vi "Auto.vi"() -> ()   [LabVIEW 2020]
uses:
  Global_Variable/Global.vi
  Global_Variable/A180648.vi
  Libraries/S7/S7.lvlib
  <userlib>/_MGI/1D Array/MGI Running Average/MGI Running Average(SGL).vi
panel:
  out "当前曲线":i16
  out "振动NHV-FFT":cluster{"f0":dbl, "df":dbl, "magnitude":dbl[]}[](graph)
  out "振动NVH-Order":cluster{"f0":dbl, "df":dbl, "magnitude":dbl[]}[](graph)
  out "试验项_Event":refnum<user-event>
  out "产品_EVENT":refnum<user-event>
  out "T1+T2":dbl
  out "T2":dbl
  out "T1":dbl
  out "吸收电流":sgl
  out "输出扭矩(大)":sgl
  out "输入扭矩":sgl
  out "当前车速":i32
  out "试验项目":T1(tab)
  out "空载试验":cluster{dbl[], dbl[]}[](graph)
  out "功能试验":cluster{dbl[], dbl[]}[](graph)
  out "力特性试验":cluster{dbl[], dbl[]}[](graph)
  out "电流特性试验":cluster{dbl[], dbl[]}[](graph)
  out "传感器特性试验":cluster{dbl[], dbl[]}[](graph)
  out "逆向空载试验":cluster{dbl[], dbl[]}[](graph)
  out "磨合":cluster{dbl[], dbl[]}[](graph)
  out "振动2NHV-FFT":cluster{"f0":dbl, "df":dbl, "magnitude":dbl[]}[](graph)
  out "振动1NVH-FFT":cluster{"f0":dbl, "df":dbl, "magnitude":dbl[]}[](graph)
  in  "判定结果":bool[][](array[boolean])=[[TRUE]]
  in  "STEP":string
  # "车速0"
  # "车速1"
  # "车速2"
  # "车速3"
  # "车速4"
  # "车速5"
  # "车速0"
  # "车速1"
  # "车速2"
  # "车速3"
  # "车速4"
  # "车速5"
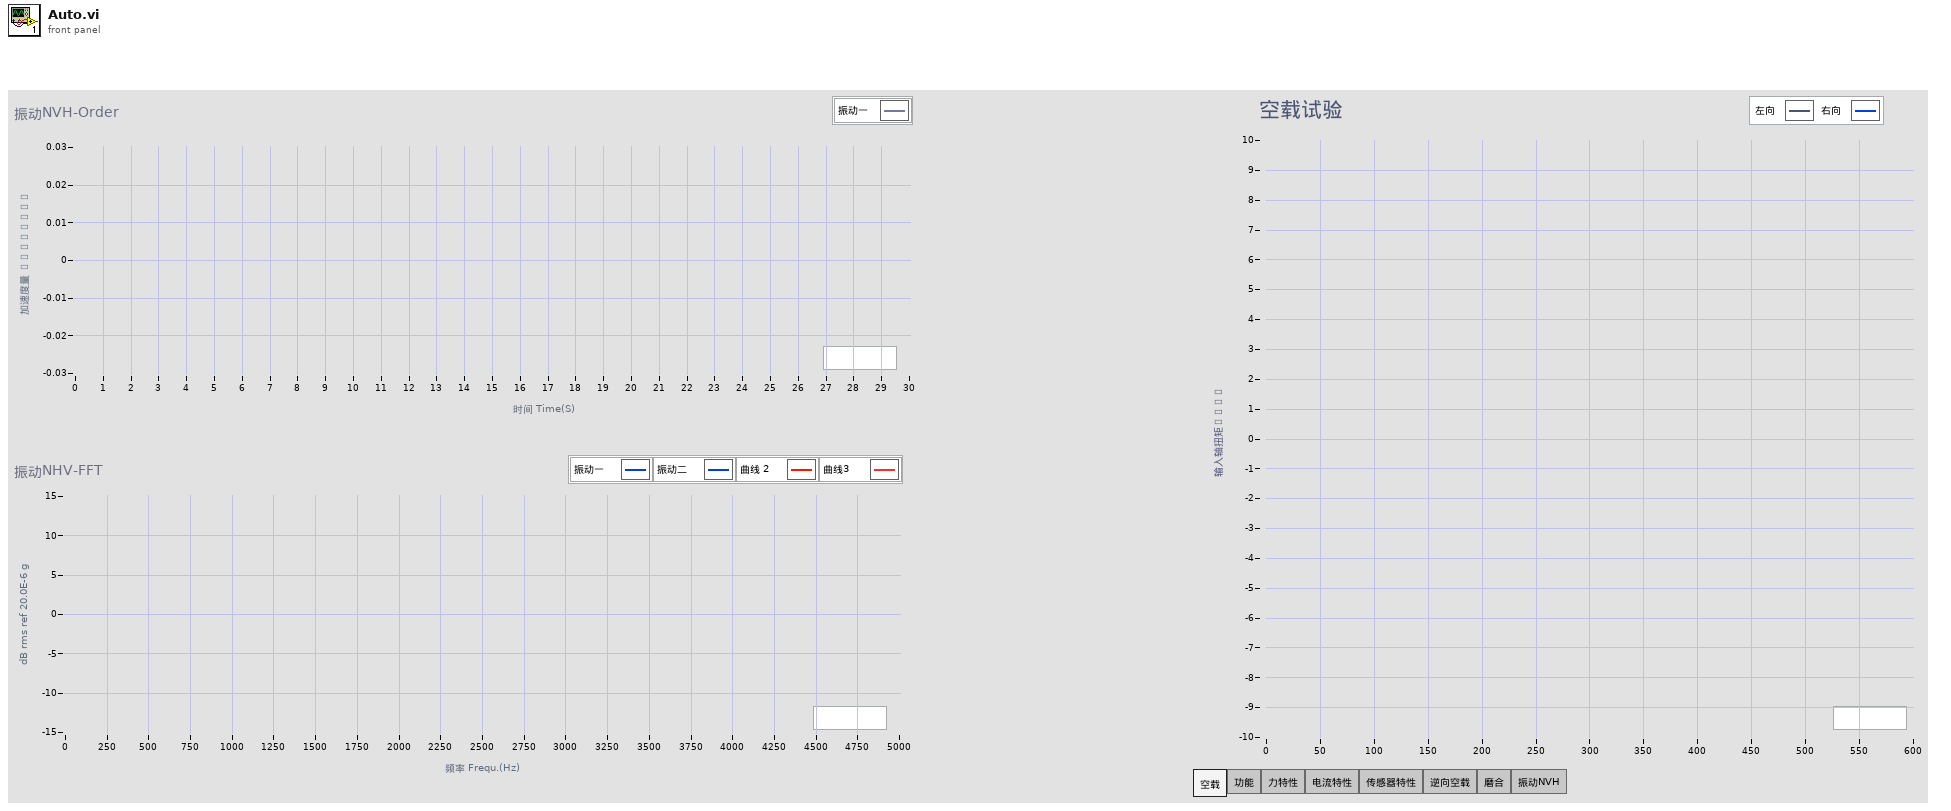
[diagram p1: front panel]
types:
  T1 = enum32{"空载", "功能", "力特性", "电流特性", "传感器特性", "逆向空载", "磨合", "振动NVH"}
  T2 = cluster{"输入轴扭矩":dbl, "输出轴扭矩小量程":dbl, "输出轴扭矩大量程":dbl}
  T3 = enum32{"空载", "功能", "力特性", "电流特性", "传感器特性", "逆向空载", "振动NVH", "磨合", "完成"}
  T4 = typedef "svc_Spectrum Info.ctl" = cluster{"channel name":string, "description":string, "x-axis units":T5, "spectral info":cluster{"spectrum type":T6, "linear/dB":enum16{"linear", "dB"}, "window":u16, "window size":i32, "FFT size":i32}, "engineering units":T7, "custom label":string, "dB reference [EU]":dbl, "peak units":enum16{"rms", "peak", "peak-peak"}, "weighting filter":T8, "spectral density?":bool, "unit label":string, "spectrum skewed?":bool, "complimentary spectrum units":T9}
  T5 = typedef "svc_X-Axis Units.ctl" = u16
  T6 = typedef "svc_Spectrum Type.ctl" = enum16{"FFT Spectrum [complex]", "Amplitude [Magnitude]", "Power [Magnitude^2]", "Cross Spectrum [complex]", "Frequency Response [Complex]"}
  T7 = typedef "svc_Engineering Units Text Ring.ctl" = u16
  T8 = typedef "svc_Weighting Filter Text Ring.ctl" = u16
  T9 = typedef "svc_Complimentary Spectrum Units.ctl" = enum16{"none", "radians", "degrees", "cycles", "imaginary"}
  T10 = cluster{"振动1频率检测段1范围":cluster{"单位":string, "下限":dbl, "上限":dbl}, "振动1频率检测段2范围":cluster{"单位":string, "下限":dbl, "上限":dbl}, "振动1频率检测段3范围":cluster{"单位":string, "下限":dbl, "上限":dbl}, "振动1频率检测段4范围":cluster{"单位":string, "下限":dbl, "上限":dbl}, "振动1频率检测段5范围":cluster{"单位":string, "下限":dbl, "上限":dbl}}
  T11 = cluster{"振动1频率检测段1振幅":cluster{"单位":string, "下限":dbl, "上限":dbl}, "振动1频率检测段2振幅":cluster{"单位":string, "下限":dbl, "上限":dbl}, "振动1频率检测段3振幅":cluster{"单位":string, "下限":dbl, "上限":dbl}, "振动1频率检测段4振幅":cluster{"单位":string, "下限":dbl, "上限":dbl}, "振动1频率检测段5振幅":cluster{"单位":string, "下限":dbl, "上限":dbl}}
  T12 = cluster{"输入旋转位移":sgl, "输入移载位移":sgl, "工装移载位移":sgl, "输入编码位移":sgl, "输入扭矩":sgl, "输出扭矩(小)":sgl, "输出扭矩(大)":sgl, "吸收电流":sgl, "Factorysensor":sgl, "输出轴旋转角度":sgl, "输出轴移栽位移":sgl, "Factorysensor2":sgl}
  T13 = typedef "lveventtype.ctl" = enum32{"Null", "Timeout", "Annotation Menu Selection", "Annotation Menu Selection?", "App Instance Close", "App Instance Close?", "Autoscale Range Change", "Bookmark Info Change", "Cell Edit", "Cell Edit?", "Cursor Grab", "Cursor Grab?", "Cursor Menu Selection", "Cursor Menu Selection?", "Cursor Move", "Cursor Release", "Data Change", "Direction Change", "Display State Change", "Drag Ended", "Drag Enter", "Drag Leave", "Drag Over", "Drag Source Update", "Drag Starting", "Drag Starting?", "Drop", "Exec State Change", "Key Down", "Key Down?", "Key Repeat", "Key Repeat?", "Key Up", "Listbox Double Click", "Menu Activation?", "Menu Selection (App)", "Menu Selection? (App)", "Menu Selection (User)", "Mouse Down", "Mouse Down?", "Mouse Enter", "Mouse Leave", "Mouse Move", "Mouse Up", "Mouse Wheel", "NI Security User Change (App)", "Pane Size", "Panel Close", "Panel Close?", "Panel Resize", "Plot Attribute Change", "Scale Range Change", "Shortcut Menu Activation?", "Shortcut Menu Selection (App)", "Shortcut Menu Selection? (App)", "Shortcut Menu Selection (User)", "Tree Double Click", "Tree Drag", "Tree Drag?", "Tree Drop", "Tree Drop?", "Tree Item Close", "Tree Item Close?", "Tree Item Open", "Tree Item Open?", "User Event", "Value Change"}
  T14 = typedef "LVPoint32TypeDef.ctl" = cluster{"Horizontal":i32, "Vertical":i32}
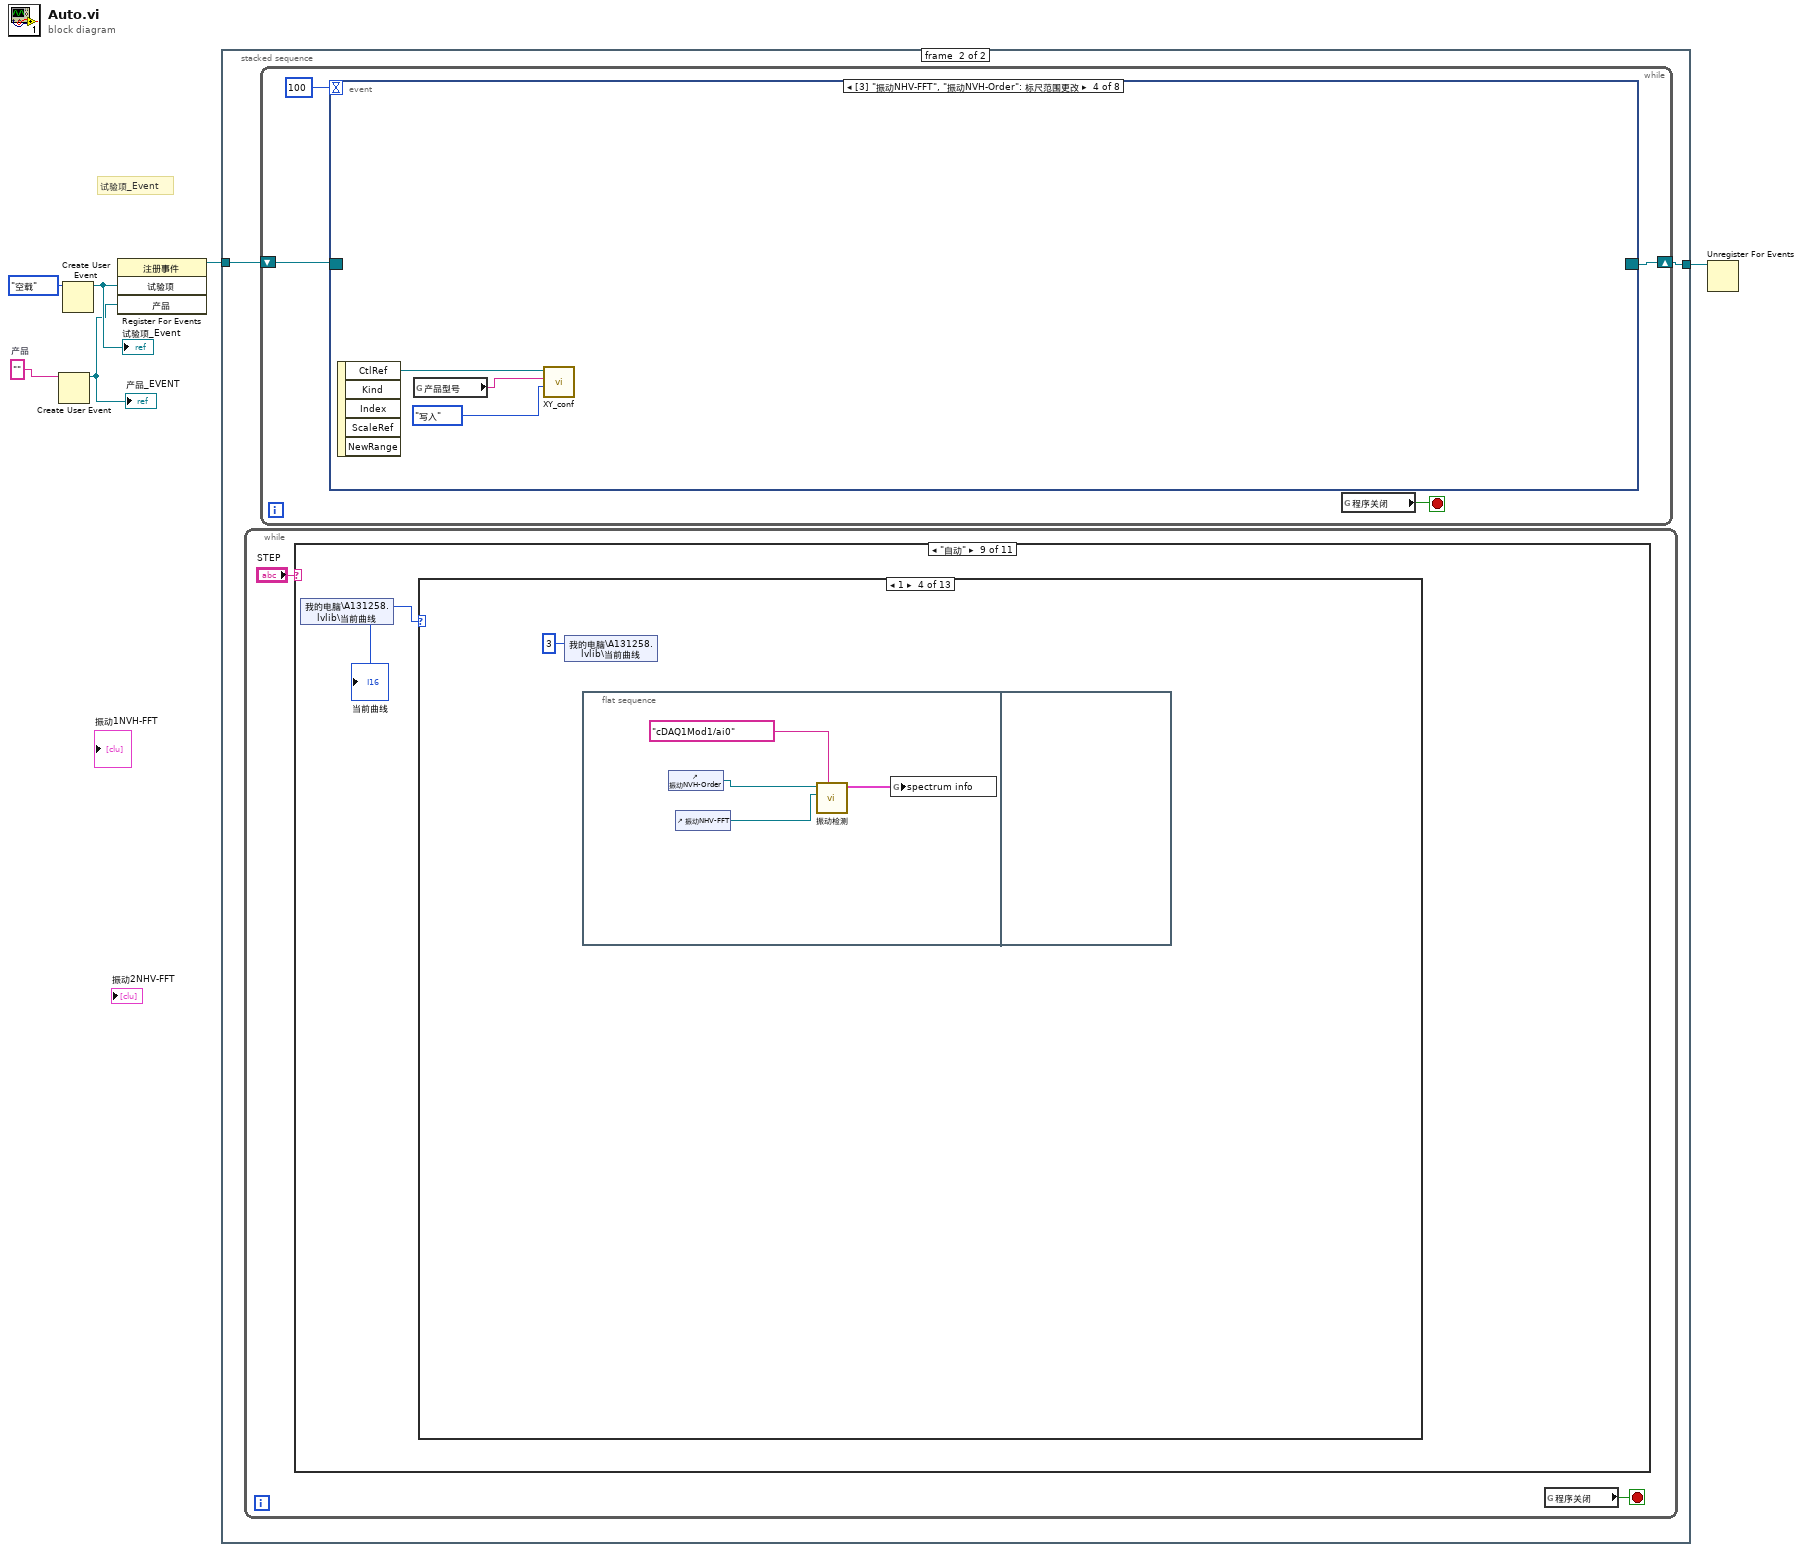
[diagram p0: block diagram]
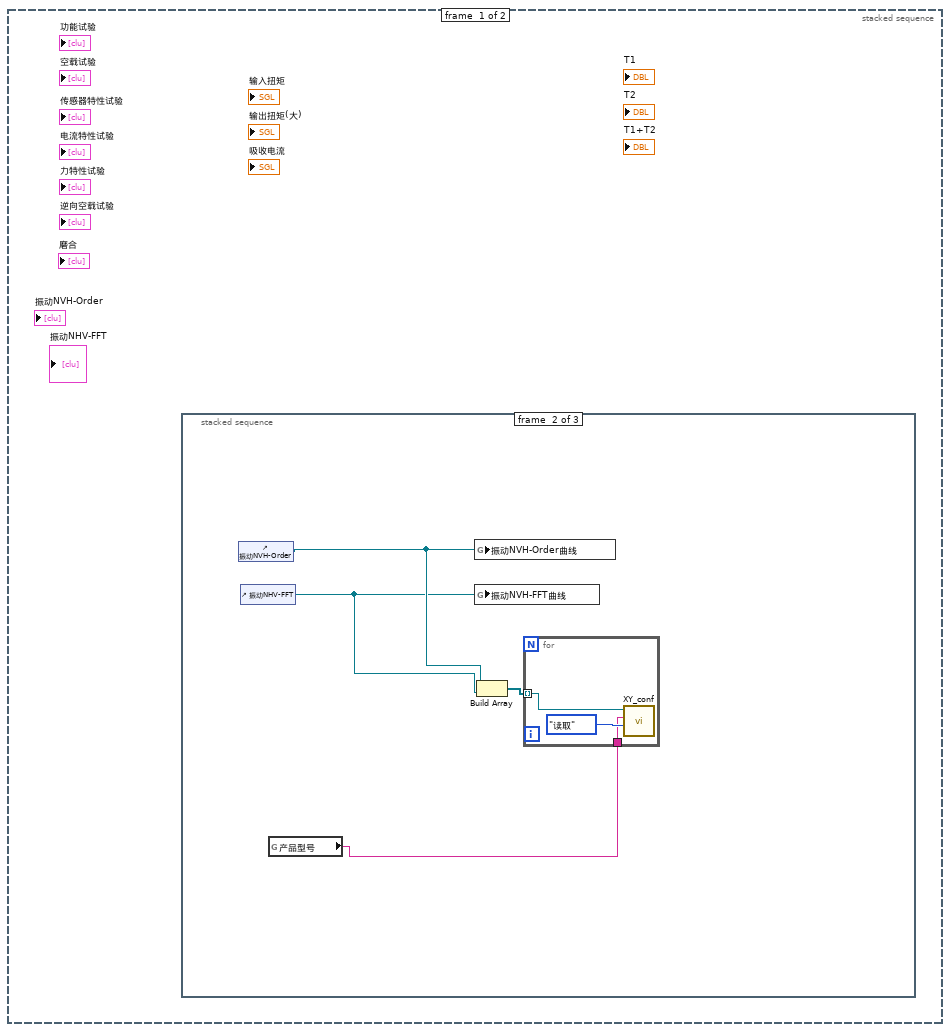
[diagram p2: hidden frame]
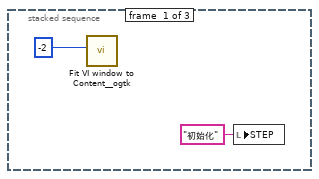
[diagram p3: hidden frame]
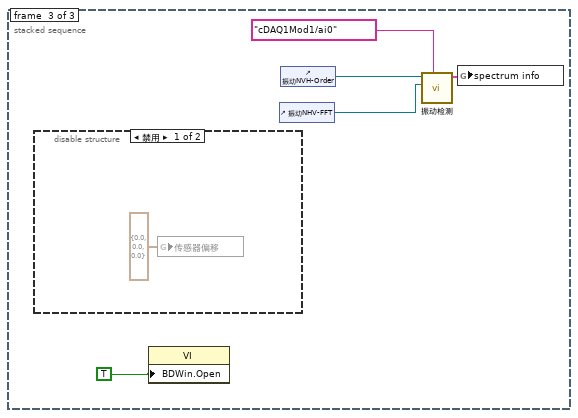
[diagram p4: hidden frame]
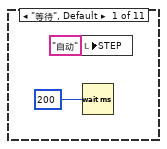
[diagram p6: hidden frame]
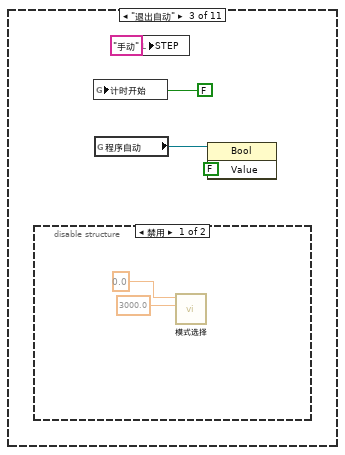
[diagram p8: hidden frame]
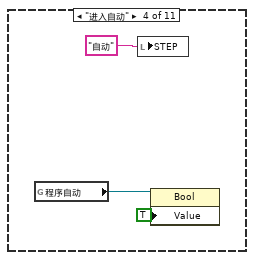
[diagram p10: hidden frame]
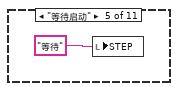
[diagram p11: hidden frame]
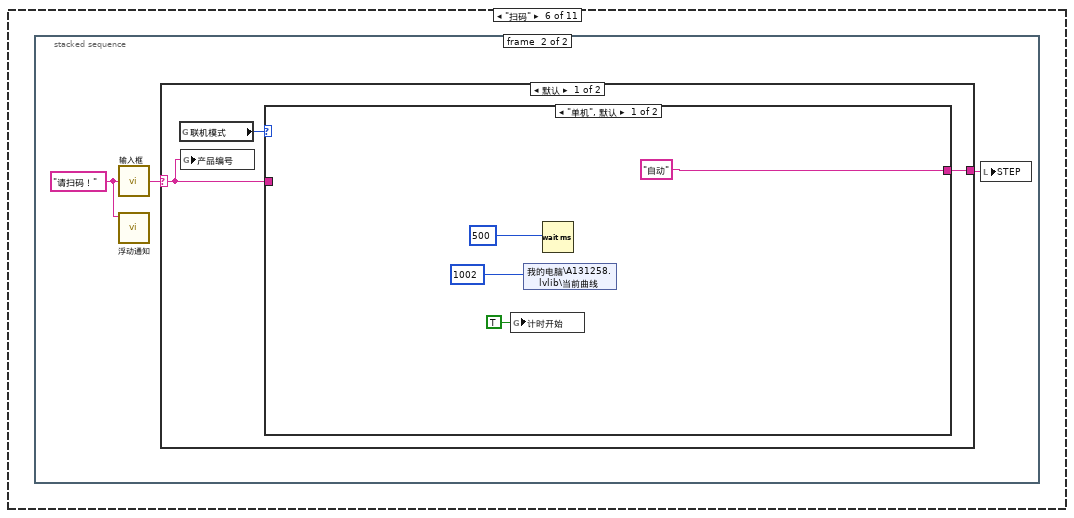
[diagram p12: hidden frame]
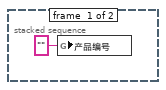
[diagram p13: hidden frame]
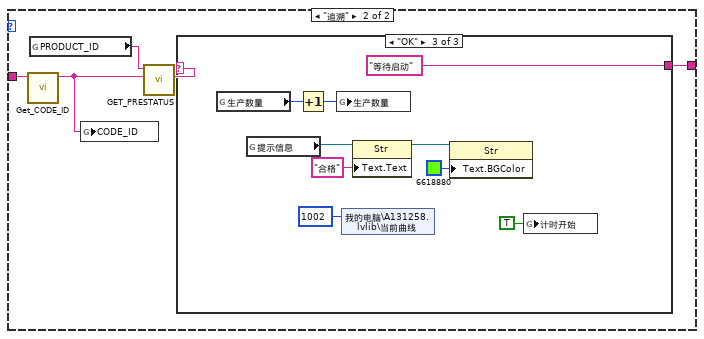
[diagram p14: hidden frame]
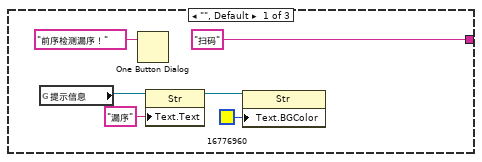
[diagram p15: hidden frame]
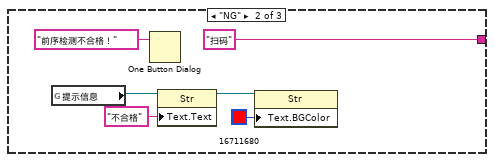
[diagram p16: hidden frame]
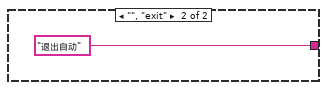
[diagram p17: hidden frame]
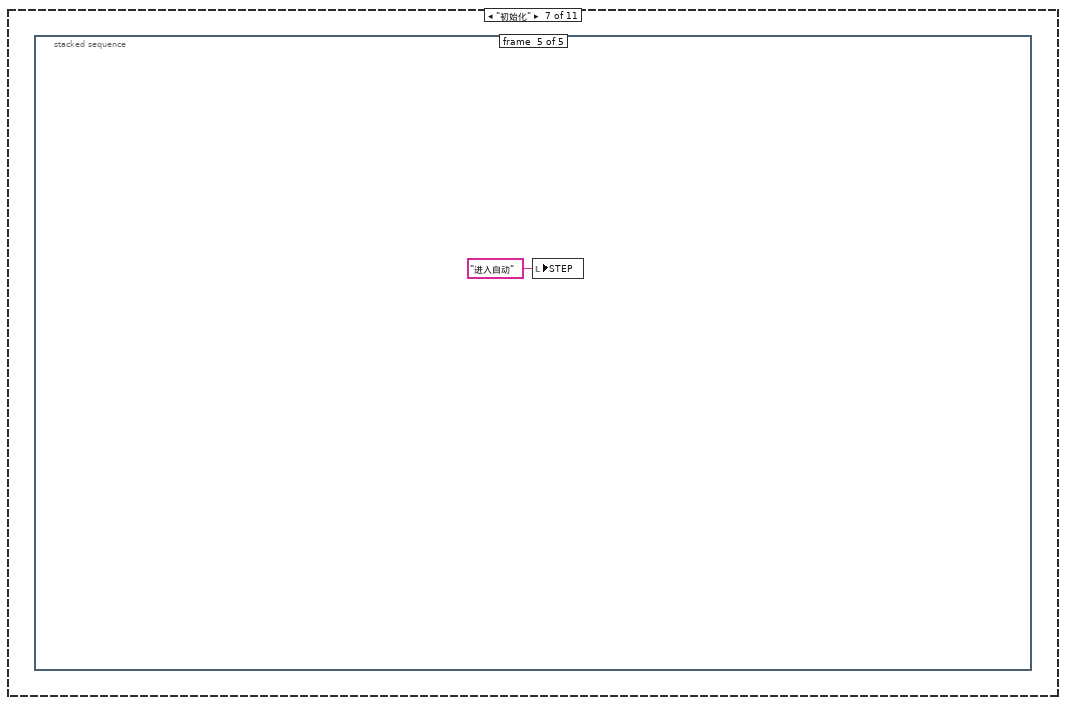
[diagram p18: hidden frame]
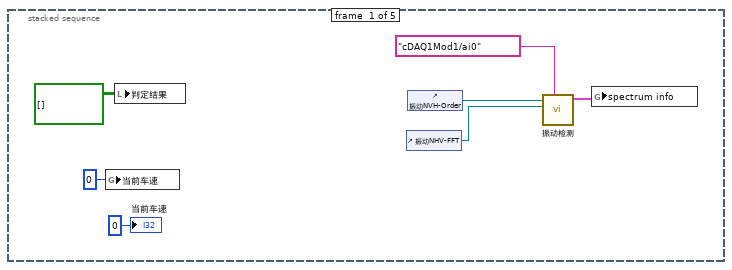
[diagram p19: hidden frame]
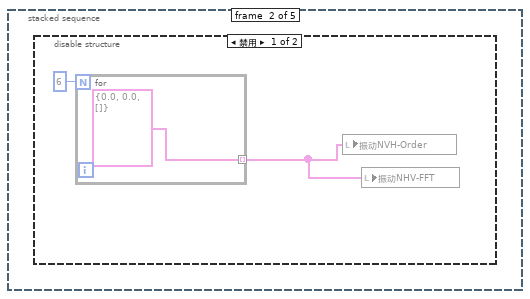
[diagram p20: hidden frame]
diagram:
  w2 = ""  # 产品
  # "试验项_Event"
  n1 = Create User Event(user event datatype=w2) -> (user event=w1:refnum<user-event>)  [unwired: 1 in, 1 out]
  "产品_EVENT" <- w1
  n2 = Create User Event(user event datatype=T1."空载" ("试验项")) -> (user event=w4:refnum<user-event>)  [unwired: 1 in, 1 out]
  "试验项_Event" <- w4
  n3 = register-events(w4, w1) -> (reference out=w5:refnum<event-registration>)  [unwired: 2 in, 1 out]
  n4 = stacked-sequence {
    tunnel: w5 -> [_ w23]
    tunnel: [_ w22] -> w3
    frame #0 {
      n5 = stacked-sequence {
        frame #0 {
          n6 = call <userlib>:"Fit VI window to Content__ogtk.vi"("border spacing (2 px)"=-2) -> ()  [unwired: 5 in, 2 out]
          n7 = local write "STEP"("初始化" ("STEP")) -> ()
        }
        frame #1 {
          n8 = control-ref of="振动NVH-Order"() -> (w10:refnum<vi>)
          n9 = control-ref of="振动NHV-FFT"() -> (w9:refnum<vi>)
          n10 = global read "Global.vi" "产品型号"() -> (w11:string)
          n11 = global write "A180648.vi" "振动NVH-Order曲线"(w10) -> ()
          n12 = global write "A180648.vi" "振动NVH-FFT曲线"(w9) -> ()
          n13 = Build Array(w10, w9) -> (w12:refnum<vi>[])
          n14 = for {
            tunnel: w12 -> [w13] mode=indexing
            tunnel: w11 -> [w14]
            n15 = call "XY_conf.vi"("方式"=enum16{"写入", "读取"}."读取", "产品"=w14, "XY图引用"=w13) -> ()  [unwired: 4 in, 1 out]
          }
        }
        frame #2 {
          n16 = disable-structure shown="禁用" {
            frame Disabled {
              n17 = global write "传感器偏移.vi" "传感器偏移"(T2 {"输入轴扭矩"=0.0, "输出轴扭矩小量程"=0.0, "输出轴扭矩大量程"=0.0} ("传感器偏移")) -> ()
            }
            frame Enabled {
            }
          }
          n18 = property class="VI"("BDWin.Open"=TRUE ("程序框图窗口:打开")) -> ()  [unwired: 2 in, 2 out]
          n19 = control-ref of="振动NHV-FFT"() -> (w17:refnum<vi>)
          n20 = control-ref of="振动NVH-Order"() -> (w18:refnum<vi>)
          n21 = call "振动检测.vi"("通道输入"=tag "cDAQ1Mod1/ai0" ("DAQmx物理通道"), "WFGraph引用句柄FFT"=w17, "WFGraph引用句柄Order"=w18) -> ("spectrum info"=w19:T4[])  [unwired: 7 in, 1 out]
          n22 = global write "Global.vi" "spectrum info"(w19) -> ()
        }
      }
    }
    frame #1 {
      n23 = while {
        stop <- w25 stop-if-true
        n24 = case shown="\"自动\"" "STEP" {
          frame "等待", Default {
            n25 = local write "STEP"("自动" ("STEP")) -> ()
            n26 = Wait (ms)(milliseconds to wait=u32 200 ("等待时间（毫秒）")) -> ()  [unwired: 1 out]
          }
          frame "手动" {
          }
          frame "退出自动" {
            n27 = disable-structure shown="禁用" {
              frame Disabled {
                n28 = call-poly "模式选择.vi"("Max Torque"=sgl 3000.0, "Velocity"=sgl 0.0) -> ()  [unwired: 9 in, 1 out]
              }
              frame Enabled {
              }
            }
            n29 = global write "Global.vi" "计时开始"(FALSE ("计时开始")) -> ()
            n30 = global read "Global.vi" "程序自动"() -> (w29:refnum<vi>)
            n31 = local write "STEP"("手动" ("STEP")) -> ()
            n32 = property class="Bool"(reference=w29, "Value"=FALSE) -> ()  [unwired: 1 in, 2 out]
          }
          frame "进入自动" {
            n33 = global read "Global.vi" "程序自动"() -> (w35:refnum<vi>)
            n34 = local write "STEP"("自动" ("STEP")) -> ()
            n35 = property class="Bool"(reference=w35, "Value"=TRUE) -> ()  [unwired: 1 in, 2 out]
          }
          frame "等待启动" {
            n36 = local write "STEP"("等待" ("STEP")) -> ()
          }
          frame "扫码" {
            n37 = stacked-sequence {
              frame #0 {
                n38 = global write "Global.vi" "产品编号"("" ("产品编号")) -> ()
              }
              frame #1 {
                w40 = "请扫码！" ("提示信息")
                n39 = call "输入框.vi"("提示信息"=w40) -> ("条形码输出"=w41:string)
                n40 = call "浮动通知.vi"("通知内容"=w40) -> ()  [unwired: 11 in]
                n41 = case shown="默认" w41 {
                  selector: w41 -> [w43 _]
                  tunnel: [w44 "退出自动" ("State(s) in Front (\"\")")] -> w39
                  frame Default {
                    n42 = global read "Global.vi" "联机模式"() -> (w42:enum16{"单机", "追溯"})
                    n43 = global write "Global.vi" "产品编号"(w43) -> ()
                    n44 = case shown="\"单机\", 默认" w42 {
                      tunnel: ["自动" ("State(s) in Front (\"\")") w53] -> w44
                      tunnel: w43 -> [_ w51]
                      frame "单机", Default {
                        n45 = global write "Global.vi" "计时开始"(TRUE ("计时开始")) -> ()
                        n46 = shared-variable "我的电脑\\A131258.lvlib\\当前曲线"(i16 1002 ("当前曲线")) -> ()  [unwired: 1 in, 1 out]
                        n47 = Wait (ms)(milliseconds to wait=u32 500 ("等待时间（毫秒）")) -> ()  [unwired: 1 out]
                      }
                      frame "追溯" {
                        n48 = call "Get_CODE_ID.vi"("CODE_SENSOR"=w51) -> ("CODE_ID"=w50:string)  [unwired: 10 in]
                        n49 = global read "追溯Global.vi" "PRODUCT_ID"() -> (w52:string)
                        n50 = global write "追溯Global.vi" "CODE_ID"(w50) -> ()
                        n51 = call "GET_PRESTATUS.vi"("CODE_ID"=w50, "PRODUCT_ID"=w52) -> ("字符串"=w49:string)  [unwired: 8 in, 1 out]
                        n52 = case shown="\"OK\"" w49 {
                          tunnel: ["扫码" ("State(s) in Front (\"\")") "扫码" ("State(s) in Front (\"\")") "等待启动" ("State(s) in Front (\"\")")] -> w53
                          frame "", Default {
                            n53 = global read "Global.vi" "提示信息"() -> (w57:refnum<vi>)
                            n54 = One Button Dialog(message="前序检测漏序！" ("消息")) -> ()  [unwired: 1 in, 1 out]
                            n55 = property class="Str"(reference=w57, "Text.Text"="漏序" ("文本.文本")) -> (reference out=w55:refnum<vi>)  [unwired: 1 in, 1 out]
                            n56 = property class="Str"(reference=w55, "Text.BGColor"=u32 16776960 ("文本.文本颜色:背景色")) -> ()  [unwired: 1 in, 2 out]
                          }
                          frame "NG" {
                            n57 = global read "Global.vi" "提示信息"() -> (w63:refnum<vi>)
                            n58 = One Button Dialog(message="前序检测不合格！" ("消息")) -> ()  [unwired: 1 in, 1 out]
                            n59 = property class="Str"(reference=w63, "Text.Text"="不合格" ("文本.文本")) -> (reference out=w61:refnum<vi>)  [unwired: 1 in, 1 out]
                            n60 = property class="Str"(reference=w61, "Text.BGColor"=u32 16711680 ("文本.文本颜色:背景色")) -> ()  [unwired: 1 in, 2 out]
                          }
                          frame "OK" {
                            n61 = global read "Global.vi" "生产数量"() -> (w72:i32)
                            n62 = global read "Global.vi" "提示信息"() -> (w71:refnum<vi>)
                            n63 = Increment(x=w72) -> (x+1=w73:i32)
                            n64 = global write "Global.vi" "生产数量"(w73) -> ()
                            n65 = shared-variable "我的电脑\\A131258.lvlib\\当前曲线"(i16 1002 ("当前曲线")) -> ()  [unwired: 1 in, 1 out]
                            n66 = property class="Str"(reference=w71, "Text.Text"="合格" ("文本.文本")) -> (reference out=w69:refnum<vi>)  [unwired: 1 in, 1 out]
                            n67 = property class="Str"(reference=w69, "Text.BGColor"=u32 6618880 ("文本.文本颜色:背景色")) -> ()  [unwired: 1 in, 2 out]
                            n68 = global write "Global.vi" "计时开始"(TRUE ("计时开始")) -> ()
                          }
                        }
                      }
                    }
                  }
                  frame "", "exit" {
                  }
                }
                n69 = local write "STEP"(w39) -> ()
              }
            }
          }
          frame "初始化" {
            n70 = stacked-sequence {
              frame #0 {
                n71 = global write "A180648.vi" "当前车速"(u16 0 ("当前车速")) -> ()
                n72 = local write "判定结果"(bool[][] [] ("判定结果")) -> ()
                n73 = control-ref of="振动NHV-FFT"() -> (w78:refnum<vi>)
                n74 = control-ref of="振动NVH-Order"() -> (w79:refnum<vi>)
                n75 = call "振动检测.vi"("通道输入"=tag "cDAQ1Mod1/ai0" ("DAQmx物理通道"), "WFGraph引用句柄FFT"=w78, "WFGraph引用句柄Order"=w79) -> ("spectrum info"=w77:T4[])  [unwired: 7 in, 1 out]
                n76 = global write "Global.vi" "spectrum info"(w77) -> ()
                "当前车速" <- 0 ("当前车速")
              }
              frame #1 {
                n77 = disable-structure shown="禁用" {
                  frame Disabled {
                    n78 = for {
                      N: 6 -> [_]
                      tunnel: [cluster{"f0":dbl, "df":dbl, "magnitude":dbl[]} {"f0"=0.0, "df"=0.0, "magnitude"=[]} ("power spectrum [dB EU]")] -> w83 mode=indexing
                    }
                    n79 = local write "振动NVH-Order"(w83) -> ()
                    n80 = local write "振动NHV-FFT"(w83) -> ()
                  }
                  frame Enabled {
                  }
                }
              }
              frame #2 {
                n81 = global read "Global.vi" "Result"() -> (w88:refnum<vi>)
                n82 = property class="Tbl"(reference=w88, "Value"=string[][] []) -> (reference out=w89:refnum<vi>, error out=w90:errorcluster)  [unwired: 1 in]
                n83 = property class="Tbl"(reference=w89, error in=w90, "Row Headers[]"=string[] [] ("列首字符串[]")) -> ()  [unwired: 2 out]
              }
              frame #3 {
                w91 = 1 ("维数大小")
                n84 = Initialize Array(" " ("字符串"), w91, w91, w91) -> (w94:string[][][])
                n85 = global write "A180648.vi" "检测结果"(w94) -> ()
                n86 = global write "A180648.vi" "当前检测项"(T3."空载" ("当前检测项")) -> ()
              }
              frame #4 {
                n87 = local write "STEP"("进入自动" ("STEP")) -> ()
              }
            }
          }
          frame "判定" {
            n88 = stacked-sequence {
              frame #0 {
                n89 = local read "振动NHV-FFT"() -> (w98:cluster{"f0":dbl, "df":dbl, "magnitude":dbl[]}[])
                n90 = global read "判定参数.vi" "振动判定范围"() -> (w110:T10)
                n91 = global read "判定参数.vi" "振动判定"() -> (w109:T11)
                n92 = global read "Global.vi" "Result"() -> (w104:refnum<vi>)
                n93 = call "振动判定.vi"("Result"=w104, "振动判定"=w109, "振动判定范围"=w110, "FFT"=w98) -> ("FFT 2"=w97:cluster{"f0":dbl, "df":dbl, "magnitude":dbl[]}[], "OK？"=w99:bool)  [unwired: 6 in]
                n94 = global read "A180648.vi" "LED-振动NVH"() -> (w105:refnum<vi>)
                n95 = local read "判定结果"() -> (w100:bool[][])
                n96 = Select(t=cluster{u32, u32}[] [{6618880, 6618880}, {6618880, 6618880}, {6618880, 6618880}, {6618880, 6618880}] ("颜色[4]"), s=w99, f=cluster{u32, u32}[] [{16711680, 16711680}, {16711680, 16711680}, {16711680, 16711680}, {16711680, 16711680}] ("颜色[4]")) -> (s? t:f=w107:cluster{u32, u32}[])
                n97 = Build Array(TRUE, w99) -> (w103:bool[])
                n98 = local write "振动NHV-FFT"(w97) -> ()
                n99 = property class="Bool"(reference=w105, "Colors [4]"=w107) -> ()  [unwired: 1 in, 2 out]
                n100 = Build Array (concatenate)(w100, w103) -> (w101:bool[][])
                n101 = local write "判定结果"(w101) -> ()
                n102 = case shown="假" w99 {
                  frame False {
                    n103 = shared-variable "我的电脑\\A131258.lvlib\\上位机测试结果"(u16 200 ("上位机测试结果")) -> ()  [unwired: 1 in, 1 out]
                  }
                  frame True {
                    n104 = shared-variable "我的电脑\\A131258.lvlib\\上位机测试结果"(u16 100 ("上位机测试结果")) -> ()  [unwired: 1 in, 1 out]
                  }
                }
                n105 = shared-variable "我的电脑\\A131258.lvlib\\当前曲线"(i16 4 ("当前曲线")) -> ()  [unwired: 1 in, 1 out]
              }
              frame #1 {
                n106 = local write "STEP"("报表" ("STEP")) -> ()
              }
            }
          }
          frame "自动" {
            n107 = shared-variable "我的电脑\\A131258.lvlib\\当前曲线"() -> (w114:i16)  [unwired: 1 in, 1 out]
            "当前曲线" <- w114
            n108 = case shown="1" w114 {
              frame -128 {
                n109 = disable-structure shown="禁用" {
                  disable-tunnel: [w118 _] -> w115
                  frame Disabled {
                    n110 = call-poly "模式选择.vi"() -> ("error out"=w118:errorcluster)  [unwired: 11 in]
                  }
                  frame Enabled {
                  }
                }
                n111 = global write "Global.vi" "计时开始"(FALSE ("计时开始")) -> ()
                n112 = disable-structure shown="禁用" {
                  disable-tunnel: w115 -> [w119 _]
                  frame Disabled {
                    n113 = call "SetActualPosition.vi"("error in (no error)"=w119) -> ()  [unwired: 10 in, 1 out]
                  }
                  frame Enabled {
                  }
                }
                n114 = call "浮动通知.vi"("通知内容"="复位中……" ("Status")) -> ()  [unwired: 11 in]
              }
              frame Default {
              }
              frame 0 {
                n115 = global write "Global.vi" "计时开始"(FALSE ("计时开始")) -> ()
                n116 = call "浮动通知.vi"("通知内容"="手动状态！" ("Status")) -> ()  [unwired: 11 in]
              }
              frame 1 {
                n117 = shared-variable "我的电脑\\A131258.lvlib\\当前曲线"(i16 3 ("当前曲线")) -> ()  [unwired: 1 in, 1 out]
                n118 = flat-sequence {
                  frame #0 {
                    n119 = control-ref of="振动NVH-Order"() -> (w124:refnum<vi>)
                    n120 = control-ref of="振动NHV-FFT"() -> (w123:refnum<vi>)
                    n121 = call "振动检测.vi"("通道输入"=tag "cDAQ1Mod1/ai0" ("DAQmx物理通道"), "WFGraph引用句柄FFT"=w123, "WFGraph引用句柄Order"=w124) -> ("spectrum info"=w126:T4[])  [unwired: 7 in, 1 out]
                    n122 = global write "Global1.vi" "spectrum info"(w126) -> ()
                  }
                  frame #1 {
                  }
                }
              }
              frame 2 {
                n123 = for {
                  N: 6 -> [_]
                  tunnel: [cluster{dbl[], dbl[]} {[], []}] -> _ mode=indexing
                  tunnel: [cluster{"f0":dbl, "df":dbl, "magnitude":dbl[]} {"f0"=0.0, "df"=0.0, "magnitude"=[]} ("power spectrum [dB EU]")] -> w133 mode=indexing
                }
                n124 = global read "Global.vi" "Result"() -> (w129:refnum<vi>)
                n125 = property class="Tbl"(reference=w129, "Value"=string[][] []) -> (reference out=w130:refnum<vi>, error out=w131:errorcluster)  [unwired: 1 in]
                n126 = local write "振动NVH-Order"(w133) -> ()
                n127 = local write "振动NHV-FFT"(w133) -> ()
                n128 = property class="Tbl"(reference=w130, error in=w131, "Row Headers[]"=string[] [] ("列首字符串[]")) -> ()  [unwired: 2 out]
              }
              frame 3 {
                n129 = local write "STEP"("判定" ("STEP")) -> ()
              }
              frame 5 {
                n130 = global write "Global.vi" "计时开始"(FALSE ("计时开始")) -> ()
              }
              frame 8 {
                n131 = call "浮动通知.vi"("通知内容"="程序停止！" ("Status")) -> ()  [unwired: 11 in]
              }
              frame 100 {
                n132 = call "浮动通知.vi"("通知内容"="请放入产品后按启动夹紧产品！" ("Status")) -> ()  [unwired: 11 in]
              }
              frame 122 {
                n133 = disable-structure shown="禁用" {
                  frame Disabled {
                    w142 = 4 ("Averaging Size")
                    n134 = call "传感器数据.vi"() -> ("传感器读数"=w149:T12)  [unwired: 10 in, 1 out]
                    n135 = Unbundle By Name(w149) -> ("输入编码位移"=w147:sgl, "输入扭矩"=w140:sgl, "输出扭矩(大)"=w144:sgl)
                    n136 = local read item#-1() -> (w141)
                    n137 = call-poly <userlib>:"MGI Running Average.vi"("Averaging Size"=w142, "Initialize? (F)"=w141, "Value"=w147) -> ("Average"=w146:sgl)  [unwired: 8 in]
                    n138 = call-poly <userlib>:"MGI Running Average.vi"("Averaging Size"=w142, "Initialize? (F)"=w141, "Value"=w140) -> ("Average"=w145:sgl)  [unwired: 8 in]
                    n139 = call-poly <userlib>:"MGI Running Average.vi"("Averaging Size"=w142, "Initialize? (F)"=w141, "Value"=w144) -> ("Average"=w143:sgl)  [unwired: 8 in]
                    n140 = Greater Or Equal To 0?(x=w146) -> (x >= 0?=w148:bool)
                    n141 = case shown="真" w148 {
                      tunnel: w145 -> [_ w167]
                      tunnel: w143 -> [_ w164]
                      tunnel: w146 -> [_ w163]
                      frame False {
                      }
                      frame True {
                        n142 = control-ref of="功能试验"() -> (w166:refnum<vi>)
                        n143 = call "曲线采集.vi"("曲线引用"=w166, "曲线索引"=0, "X"=w163, "Y"=w167) -> ("错误输出"=w162:errorcluster)  [unwired: 10 in, 1 out]
                        n144 = call "曲线采集.vi"("曲线引用"=w166, "曲线索引"=2, "X"=w163, "Y"=w164) -> ()  [unwired: 10 in, 2 out]
                        n145 = Unbundle By Name(w162) -> ("status"=w161:bool)
                        n146 = local write item#-1(w161) -> ()
                      }
                    }
                    n147 = case shown="真" w141 {
                      frame False {
                      }
                      frame True {
                        n148 = control-ref of="振动1NVH-FFT"() -> (w151:refnum<vi>)
                        n149 = control-ref of="振动2NHV-FFT"() -> (w150:refnum<vi>)
                        n150 = vi-ref "NVH_TEST.vi"() -> (w152:refnum<vi>)
                        n151 = property class="VI"(reference=w152) -> (error out=w156:errorcluster, "Name"=w157:string)  [unwired: 1 in, 1 out]
                        n152 = Open VI Reference(type specifier VI Refnum (for type only)=refnum<vi> refnum, vi path=w157, options=128 ("调用并忽略输出"), error in (no error)=w156) -> (vi reference=w154:refnum<vi>)  [unwired: 2 in, 1 out]
                        n153 = call-by-ref "开始异步调用"(reference=w154, "振动NHV-FFT"=w150, "振动NVH-Order"=w151) -> (reference out=w160:refnum<vi>, error out=w158:errorcluster)  [unwired: 11 in]
                        n154 = Close Reference(reference=w160, error in (no error)=w158) -> (error out=w159:errorcluster)
                        n155 = call <vilib>:"Simple Error Handler.vi"("error in (no error)"=w159) -> ()  [unwired: 4 in, 5 out]
                      }
                    }
                  }
                  frame Enabled {
                  }
                }
              }
              frame 999 {
                n156 = call "浮动通知.vi"("通知内容"="请启动！" ("Status")) -> ()  [unwired: 11 in]
              }
              frame 1002 {
                n157 = call "浮动通知.vi"("通知内容"="请启动！" ("Status")) -> ()  [unwired: 11 in]
              }
              frame 1000 {
                n158 = local write "STEP"("扫码" ("STEP")) -> ()
              }
            }
          }
          frame "合格判定" {
            n159 = Wait (ms)(milliseconds to wait=u32 100 ("等待时间（毫秒）")) -> ()  [unwired: 1 out]
            n160 = local write "STEP"("等待" ("STEP")) -> ()
          }
          frame "报表" {
            n161 = stacked-sequence {
              frame #0 {
                n162 = global write "Global.vi" "计时开始"(FALSE ("计时开始")) -> ()
                n163 = shared-variable "我的电脑\\A131258.lvlib\\当前曲线"(i16 5 ("当前曲线")) -> ()  [unwired: 1 in, 1 out]
              }
              frame #1 {
                n164 = global read "Global.vi" "产品编号"() -> (w180:string)
                n165 = call "Report.vi"("文件重命名"=TRUE, "文件名称"=w180, "检测结果"="判定结果") -> ("error out"=w179:errorcluster, "PRODUCT_VAULE"=w177:string)  [unwired: 7 in]
                n166 = global read "Global.vi" "联机模式"() -> (w182:enum16{"单机", "追溯"})
                n167 = call <vilib>:"Simple Error Handler.vi"("error in (no error)"=w179) -> ("error out"=w176:errorcluster)  [unwired: 4 in, 4 out]
                n168 = case shown="\"追溯\"" w182 {
                  tunnel: w177 -> [_ w184]
                  tunnel: w176 -> [_ w183]
                  frame "单机", Default {
                  }
                  frame "追溯" {
                    n169 = global read "追溯Global.vi" "DEVICE_ID"() -> (w193:string)
                    n170 = global read "追溯Global.vi" "CODE_ID"() -> (w194:string)
                    n171 = global read "追溯Global.vi" "USER_ID"() -> (w192:string)
                    n172 = global read "Global.vi" "Result"() -> (w186:refnum<vi>)
                    n173 = call "UPRESULT.vi"("DEVICE_ID"=w193, "USER_ID"=w192, "CODE_ID"=w194, "RESULT_VALUE"=w184, "错误输入"=w183) -> ()  [unwired: 10 in, 1 out]
                    n174 = property class="Tbl"(reference=w186) -> (reference out=w191:refnum<vi>, error out=w188:errorcluster, "Row Headers[]"=w189:string[])  [unwired: 1 in]
                    n175 = property class="Tbl"(reference=w191, error in=w188) -> (error out=w187:errorcluster, "Value"=w190:string[][])  [unwired: 1 out]
                    n176 = for {
                      tunnel: w190 -> [w198] mode=indexing
                      tunnel: w189 -> [w199] mode=indexing
                      tunnel: [w196] -> w185 mode=indexing if=w197
                      shift-right: [w195] -> _
                      shift-left: w187 -> [w195]
                      n177 = Build Array (concatenate)(w199, w198) -> (w196:string[])
                      n178 = Index Array(array=w198) -> (element=w200:string)  [unwired: 1 in]
                      n179 = case shown="默认" w200 {
                        tunnel: [TRUE FALSE] -> w197
                        frame Default {
                        }
                        frame "" {
                        }
                      }
                    }
                    n180 = call "UPTEST.vi"("Result"=w185, "CODE_ID"=w194, "DEVICE_ID"=w193) -> ()  [unwired: 6 in, 1 out]
                  }
                }
              }
              frame #2 {
                n181 = local write "STEP"("进入自动" ("STEP")) -> ()
              }
            }
          }
        }
        n182 = global read "Global.vi" "程序关闭"() -> (w25:bool)
      }
      n183 = while {
        shift-right: [w204] -> w22
        shift-left: w23 -> [w205]
        stop <- w206 stop-if-true
        n184 = event shown="[3] \"振动NHV-FFT\", \"振动NVH-Order\": 标尺范围更改" {
          selector: w205 -> [_ _ _ _ _ _ _ _]
          dyn-events: [_ _ _ _ _ _ _ _] -> w204
          timeout: 100 -> [_ _ _ _ _ _ _ _]
          event Timeout {
            n185 = event-data() -> ()  [unwired: 1 in, 3 out]
            n186 = disable-structure shown="禁用" {
              frame Disabled {
                n187 = call "Obtain Broadcast Events for Registration.vi"() -> ("Already running?"=w208:bool)  [unwired: 9 in, 2 out]
                n188 = case shown="真" w208 {
                  frame False {
                    n189 = local write "STEP"("手动" ("STEP")) -> ()
                  }
                  frame True {
                    n190 = call "错误代码.vi"() -> ("Status_Read"=w210:u32)  [unwired: 11 in]
                    n191 = feedback #1() -> (w220:u32)  [unwired: 1 in]
                    n192 = feedback-in #1(w210) -> ()
                    n193 = case shown="1, 默认" w210 {
                      frame 0 {
                        n194 = global read "Global.vi" "报警图标"() -> (w221:refnum<vi>)
                        n195 = property class="Bool"(reference=w221, "Visible"=FALSE ("可见")) -> ()  [unwired: 1 in, 2 out]
                      }
                      frame 1, Default {
                        n196 = global read "Global.vi" "报警图标"() -> (w224:refnum<vi>)
                        n197 = property class="Bool"(reference=w224, "Visible"=TRUE ("可见")) -> ()  [unwired: 1 in, 2 out]
                      }
                    }
                    n198 = Greater Or Equal?(x=w210, y=i16 5000) -> (x >= y?=w218:bool)
                    n199 = Less?(x=w210, y=i16 5200) -> (x < y?=w219:bool)
                    n200 = Equal?(x=w210, y=w220) -> (x = y?=w217:bool)
                    n201 = global read "Global.vi" "报警图标"() -> (w212:refnum<vi>)
                    n202 = And(x=w218, y=w219) -> (x .and. y?=w211:bool)
                    n203 = property class="Bool"(reference=w212, "Value"=w211) -> ()  [unwired: 1 in, 2 out]
                    n204 = Bundle By Name(cluster=errorcluster {"status"=FALSE, "code"=0, "source"=""} ("错误常量"), "status"=w211, "code"=w210) -> (w216:errorcluster)
                    n205 = case shown="假" w217 {
                      tunnel: w216 -> [w225 _]
                      frame False {
                        n206 = call "报警处理.vi"("错误常量"=w225) -> ()  [unwired: 9 in, 2 out]
                      }
                      frame True {
                      }
                    }
                  }
                }
              }
              frame Enabled {
              }
            }
          }
          event User Event {
            n207 = event-data() -> ("试验项"=w226:T1)  [unwired: 1 in]
            "试验项目" <- w226
            n208 = disable-structure shown="禁用" {
              disable-tunnel: w226 -> [w227 _]
              frame Disabled {
                n209 = global read "A180648.vi" "检测结果"() -> (w230:string[][][])
                n210 = global read "Global.vi" "Result"() -> (w228:refnum<vi>)
                n211 = Index Array(array=w230, index (dim 0)=w227) -> (element=w229:string[][])  [unwired: 2 in]
                n212 = property class="Tbl"(reference=w228, "Value"=w229) -> ()  [unwired: 1 in, 2 out]
              }
              frame Enabled {
              }
            }
          }
          event "试验项目": Value Change {
            n213 = event-data() -> ("NewVal"=w231:T1)  [unwired: 1 in]
            n214 = disable-structure shown="禁用" {
              disable-tunnel: w231 -> [w235 _]
              frame Disabled {
                n215 = global read "A180648.vi" "检测结果"() -> (w234:string[][][])
                n216 = global read "Global.vi" "Result"() -> (w232:refnum<vi>)
                n217 = Index Array(array=w234, index (dim 0)=w235) -> (element=w233:string[][])  [unwired: 2 in]
                n218 = property class="Tbl"(reference=w232, "Value"=w233) -> ()  [unwired: 1 in, 2 out]
              }
              frame Enabled {
              }
            }
          }
          event "振动NHV-FFT", "振动NVH-Order": Scale Range Change {
            n219 = event-data() -> ("CtlRef"=w237:refnum<vi>)  [unwired: 1 in, 4 out]
            n220 = global read "Global.vi" "产品型号"() -> (w236:string)
            n221 = call "XY_conf.vi"("方式"=enum16{"写入", "读取"}."写入", "产品"=w236, "XY图引用"=w237) -> ()  [unwired: 4 in, 1 out]
          }
          event User Event {
            n222 = event-data() -> ("产品"=w241:string)  [unwired: 1 in]
            n223 = control-ref of="振动NHV-FFT"() -> (w239:refnum<vi>)
            n224 = control-ref of="振动NVH-Order"() -> (w240:refnum<vi>)
            n225 = Build Array(w240, w239) -> (w242:refnum<vi>[])
            n226 = for {
              tunnel: w242 -> [w243] mode=indexing
              tunnel: w241 -> [w244]
              n227 = call "XY_conf.vi"("方式"=enum16{"写入", "读取"}."读取", "产品"=w244, "XY图引用"=w243) -> ()  [unwired: 4 in, 1 out]
            }
          }
          event Panel Close {
            n228 = event-data() -> ()  [unwired: 1 in, 4 out]
            n229 = global write "Global.vi" "程序关闭"(TRUE ("程序关闭")) -> ()
          }
          event "电流特性试验", "传感器特性试验", "力特性试验", "空载试验", "功能试验", "逆向空载试验": Mouse Enter; "电流特性试验", "传感器特性试验", "力特性试验", "空载试验", "功能试验", "逆向空载试验": Mouse Leave; "电流特性试验", "传感器特性试验", "力特性试验", "空载试验", "功能试验", "逆向空载试验": Cursor Move {
            n230 = event-data() -> ("CtlRef"=w249:refnum<vi>, "Type"=w247:T13)  [unwired: 1 in]
            n231 = call "CursorShow.vi"("nameShow"=TRUE, "Type"=w247, "Graph"=w249) -> ()  [unwired: 7 in, 2 out]
          }
          event "电流特性试验", "传感器特性试验", "力特性试验", "空载试验", "功能试验", "逆向空载试验", "磨合": Mouse Down {
            n232 = event-data() -> ("CtlRef"=w254:refnum<vi>, "Coords"=w253:T14, "Type"=w251:T13)  [unwired: 1 in]
            n233 = invoke class="XYGraph (严格)" method="Map Coords To XY"(reference=w254, "Coords"=w253) -> (reference out=w252:refnum<vi>, "XY"=w250:cluster{"X":dbl, "Y":dbl})  [unwired: 5 in, 5 out]
            n234 = call "CursorShow.vi"("游标.游标位置"=w250, "Type"=w251, "Graph"=w252) -> ()  [unwired: 7 in, 2 out]
          }
        }
        n235 = global read "Global.vi" "程序关闭"() -> (w206:bool)
      }
    }
  }
  n236 = Unregister For Events(event registration refnum=w3) -> ()  [unwired: 1 in, 1 out]
